vi "CreateDirectoryIfNone.vi"(8 "error in":errorcluster, 11 "path":path) -> (0 "error out":errorcluster)   [LabVIEW 2013]
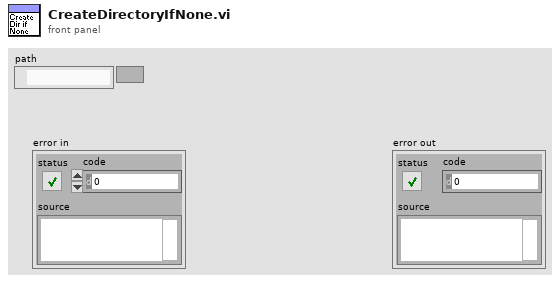
[diagram p1: front panel]
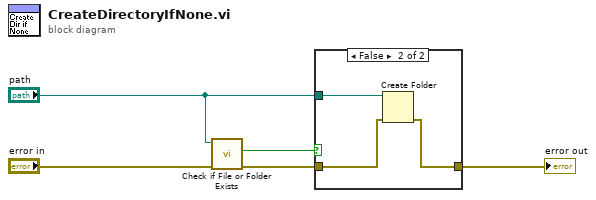
[diagram p0: block diagram]
diagram:
  n1 = call <vilib>:"Check if File or Folder Exists.vi"("error in (no error)"="error in", "path"="path") -> ("error out"=w2:errorcluster, "file or folder exists?"=w4:bool)  [unwired: 7 in, 1 out]
  n2 = case shown="False" w4 {
    tunnel: [w6 w7] -> w5
    tunnel: w2 -> [w6 w8]
    tunnel: "path" -> [_ w9]
    frame True {
    }
    frame False {
      n3 = Create Folder(path (use dialog)=w9, error in=w8) -> (error out=w7:errorcluster)  [unwired: 1 in, 2 out]
    }
  }
  "error out" <- w5
